vi "Launch Nested.vi"(8 "error in (no error)":errorcluster, 9 "Actor":refnum<class "Actor.lvclass">, 10 "Name":string, 11 "MVVM Abstruct View in":refnum<class "MVVM Abstruct View.lvclass">) -> (0 "error out":errorcluster, 3 "MVVM Abstruct View out":refnum<class "MVVM Abstruct View.lvclass">)   [LabVIEW 2020, in "MVVM Abstruct View.lvlib" / "MVVM Abstruct View.lvclass"]
uses:
  MVVM Abstruct View.lvclass
  C:/Program Files (x86)/National Instruments/LabVIEW 2020/vi.lib/ActorFramework/Actor/Actor.lvclass
  <vilib>/ActorFramework/Actor/Actor.lvclass
  <vilib>/ActorFramework/Message/Message.lvclass
  MVVM Abstruct View.lvclass/MVVM Abstruct View.ctl
  <vilib>/ActorFramework/Actor/Actor.lvclass/Actor.ctl
  <vilib>/ActorFramework/Message Enqueuer/Message Enqueuer.lvclass/Message Enqueuer.ctl
  Enqueues Data/Enqueues Data.lvclass
  Enqueues Data/Enqueues Data.lvclass/Enqueues Data.ctl
  MVVM Abstruct Controller/MVVM Abstruct Controller Messages/Add & Register Views Msg/Add & Register Views Msg.lvclass/Add & Register Views Msg.ctl
  Enqueues Data/Accessors/Write ActorMap.vi
  MVVM Abstruct Controller/MVVM Abstruct Controller Messages/Add & Register Views Msg/Add & Register Views Msg.lvclass
  C:/Program Files (x86)/National Instruments/LabVIEW 2020/vi.lib/ActorFramework/Message/Message.lvclass
  <vilib>/ActorFramework/Message Priority Queue/Priority Enqueue.vi
  C:/Users/yu/Desktop/Pro1/06 Source/Code/Common/ActorMap/ActorMap.lvclass
  <vilib>/ActorFramework/Message Enqueuer/Message Enqueuer.lvclass
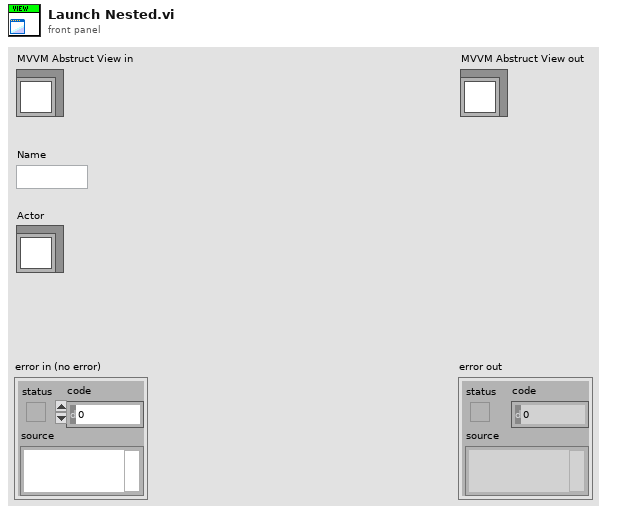
[diagram p1: front panel]
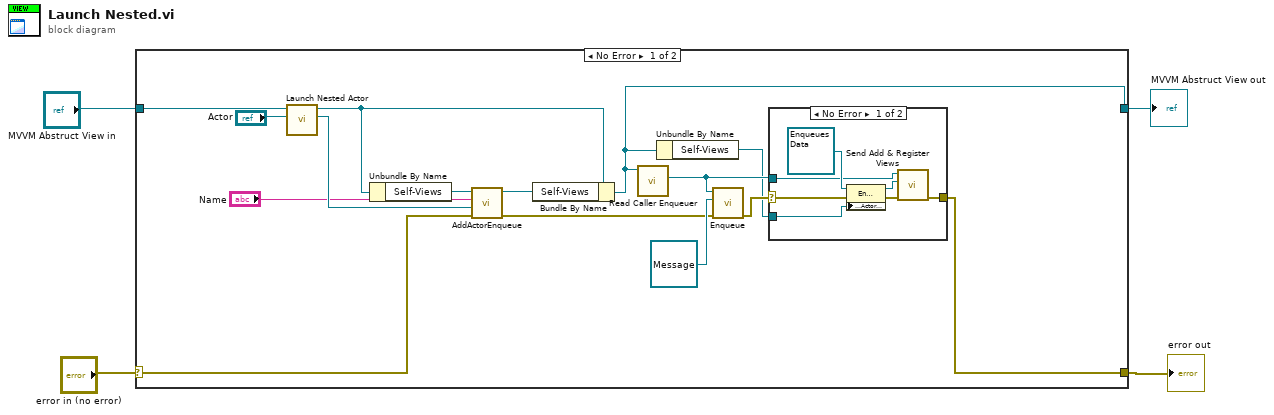
[diagram p0: block diagram]
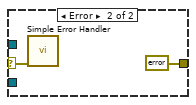
[diagram p2: hidden frame]
diagram:
  n1 = case shown="No Error" "error in (no error)" {
    selector: "error in (no error)" -> [w12 w30]
    tunnel: [w8 w30] -> w1
    tunnel: [w6 w29] -> w3
    tunnel: "MVVM Abstruct View in" -> [w19 w29]
    frame No Error {
      n2 = call <vilib>:"Launch Nested Actor.vi"("Nested Actor"="Actor", "Caller Actor in"=w19) -> ("Nested Actor's Enqueuer"=w14:refnum<class "Message Enqueuer.lvclass">, "Caller Actor out"=w17:refnum<class "MVVM Abstruct View.lvclass">)  [unwired: 7 in, 1 out]
      n3 = Unbundle By Name(w17) -> ("Self-Views"=w16:refnum<class "ActorMap.lvclass">)
      n4 = call "AddActorEnqueue.vi"("error in (no error)"=w12, "Actor's Enqueuer"=w14, "name"="Name", "ActorMap in"=w16) -> ("error out"=w9:errorcluster, "ActorMap out"=w15:refnum<class "ActorMap.lvclass">)  [unwired: 6 in]
      n5 = Bundle By Name(cluster=w17, "Self-Views"=w15) -> (w6:refnum<class "MVVM Abstruct View.lvclass">)
      n6 = call <vilib>:"Read Caller Enqueuer.vi"("Actor"=w6) -> ("Caller Enqueuer"=w7:refnum<class "Message Enqueuer.lvclass">)  [unwired: 10 in]
      n7 = Unbundle By Name(w6) -> ("Self-Views"=w5:refnum<class "ActorMap.lvclass">)
      n8 = call <vilib>:"Enqueue.vi"("error in (no error)"=w9, "Message"=refnum<class "Message.lvclass"> refnum, "Message Enqueuer in"=w7) -> ("error out"=w10:errorcluster)  [unwired: 7 in, 1 out]
      n9 = case shown="No Error" w10 {
        selector: w10 -> [w20 w28]
        tunnel: [w23 errorcluster {"status"=FALSE, "code"=0, "source"=""} ("error out")] -> w8
        tunnel: w7 -> [w22 _]
        tunnel: w5 -> [w25 _]
        frame No Error {
          n10 = property class="Enqueues Data.lvclass"(reference=refnum<class "Enqueues Data.lvclass"> refnum ("View"), error in=w20, "Accessors:ActorMap"=w25) -> (reference out=w24:refnum<class "Enqueues Data.lvclass">, error out=w21:errorcluster)
          n11 = call "Send Add & Register Views.vi"("error in (no error)"=w21, "View"=w24, "Message Enqueuer"=w22) -> ("error out"=w23:errorcluster)  [unwired: 7 in, 1 out]
        }
        frame Error {
          n12 = call <vilib>:"Simple Error Handler.vi"("error in (no error)"=w28) -> ()  [unwired: 4 in, 5 out]
        }
      }
    }
    frame Error {
    }
  }
  "error out" <- w1
  "MVVM Abstruct View out" <- w3
